vi "test.vi"() -> ()   [LabVIEW 2011]
panel:
  out "Boolean":bool
  in  "Play Button":bool
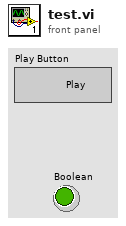
[diagram p1: front panel]
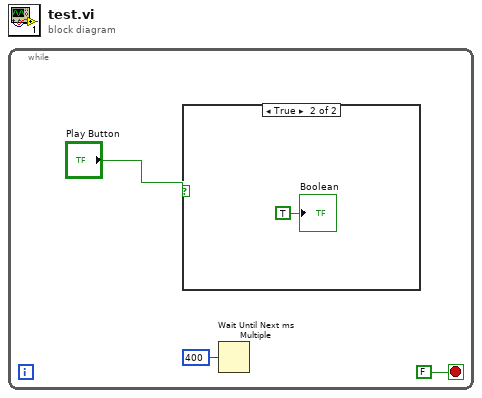
[diagram p0: block diagram]
diagram:
  n1 = while {
    stop <- FALSE stop-if-true
    n2 = case shown="True" "Play Button" {
      frame False {
      }
      frame True {
        "Boolean" <- TRUE ("Boolean")
      }
    }
    n3 = Wait Until Next ms Multiple(millisecond multiple=u32 400) -> ()  [unwired: 1 out]
  }
